vi "Edge Detection Comparizon.vi"() -> ()   [LabVIEW 2023]
doc: "This example shows the application of the wavelet transforms in detecting image edges.\n\nConventional edge detection methods process an image at a single resolution and return a binary edge map. The wavelet transform-based method processes an image at multiple levels of resolution and returns a series of grey-level edge maps at different resolutions. You can obtain the global profile of the image in a low-resolution edge map and the detailed texture of the image in a high-resolution edge map.\n\nThis example uses the WA Multiscale Edge Detection VI to detect the edges of an image.\n\n<b>Instructions:</b>\n1) Run this VI.\n2) Increase the value of <b>Level</b> to observe coarser edges.\n3) Increase the value of <b>Threshold Ratio</b> to skip the edges in darker areas."
uses:
  Images/_Images.ctl
  <vilib>/vision/NI_Vision_Development_Module.lvlib
panel:
  out "Edges 2":T1(plugin-control)
  in  "Threshold Value":sgl format="%.2f"
  in  "Method":T2(ring)
  out "error out":errorcluster
  in  "error in (no error)":errorcluster
  in  "Image":T3
  in  "wavelet":u16(ring)=20 items=["db02"=0, "db03"=1, "db04"=2, "db05"=3, "db06"=4, "db07"=5, "db08"=6, "db09"=7, "db10"=8, "db11"=9, "db12"=10, "db13"=11, "db14"=12, "Haar"=13, "bior1_3"=14, "bior1_5"=15, "bior2_2"=16, "bior2_4"=17, "bior2_6"=18, "bior2_8"=19, "bior3_1"=20, "bior3_3"=21, "bior3_5"=22, "bior3_7"=23, "bior3_9"=24, "bior4_4 (FBI)"=25, "bior5_5"=38, "bior6_8"=39, "coif1"=26, "coif2"=27, "coif3"=28, "coif4"=29, "coif5"=30, "sym2"=31, "sym3"=32, "sym4"=33, "sym5"=34, "sym6"=35, "sym7"=36, "sym8"=37]
  out "Edges":T1(plugin-control)
  out "Source Image":T1(plugin-control)
  in  "Level":i32=1 min=1 max=8
  in  "Threshold ratio":dbl=0.1 min=0.0001 max=1.0 step=0.1
  # "Edges detection using Wavelets"
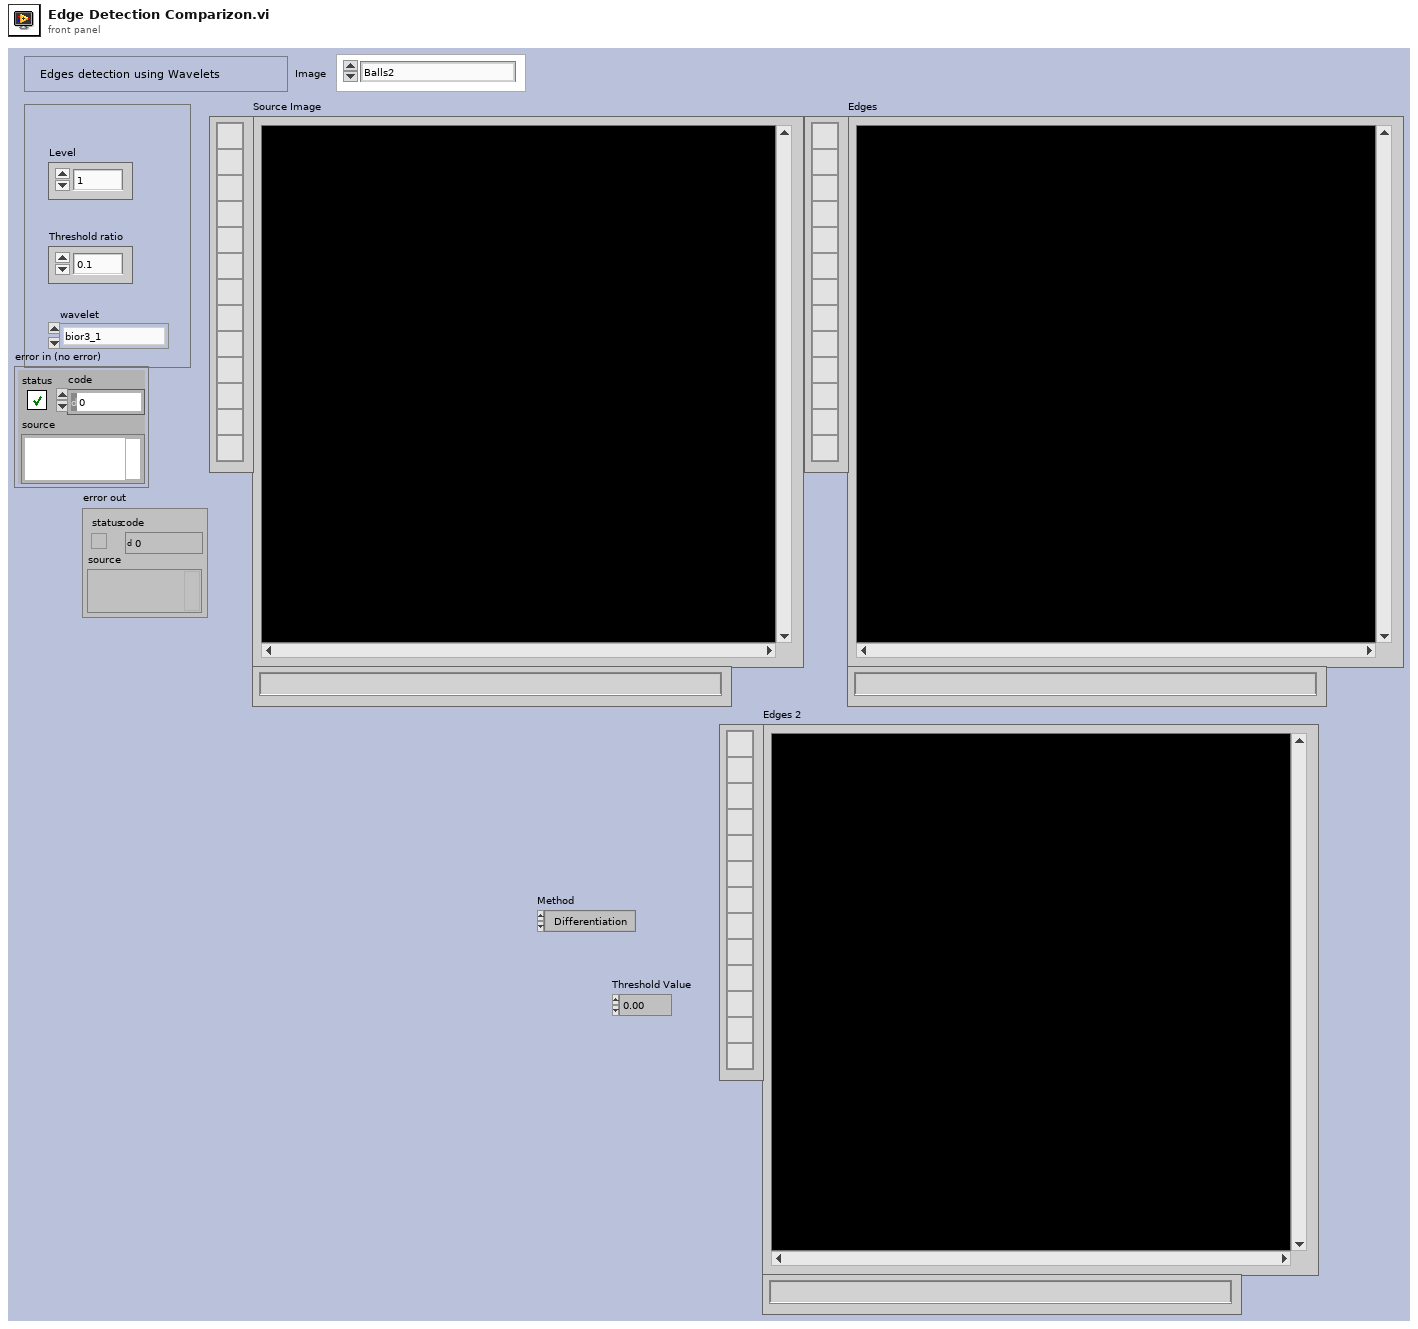
[diagram p1: front panel]
types:
  T1 = typedef "IMAQ Image.ctl" = refnum<image>
  T2 = enum32{"Differentiation", "Gradient", "Prewitt", "Roberts", "Sigma", "Sobel"}
  T3 = typedef "_Images.ctl" = enum16{"Balls2", "Battery1", "Battery2", "Connector1", "Subwoofer1", "Subwoofer2", "Subwoofer3", "Subwoofer4", "Hase1", "Lamp1", "Lamp2", "Mouse1", "PhotoLens1", "Po1", "PowerSupply1", "Router", "--- Step Wedges ---", "Stepwedge1", "Stepwedge2", "Stepwedge3", "--- Fusion ---", "Fusion160kV", "Fusion2-120kV", "Fusion2-320kV", "Fusion300kV", "FusionPart1-120kV", "FusionPart1-180kV", "--- PART 01 ---", "Part1", "Part2", "Part3", "Part4", "Part5", "Part6", "Part7", "Part8", "--- Different Integrations ---", "Step2737-02Int", "Step2737-04Int", "Step2737-08Int", "Step2737-16Int", "Step2737-32Int", "Step2737-64Int"}
  T4 = typedef "Image Type" = u32
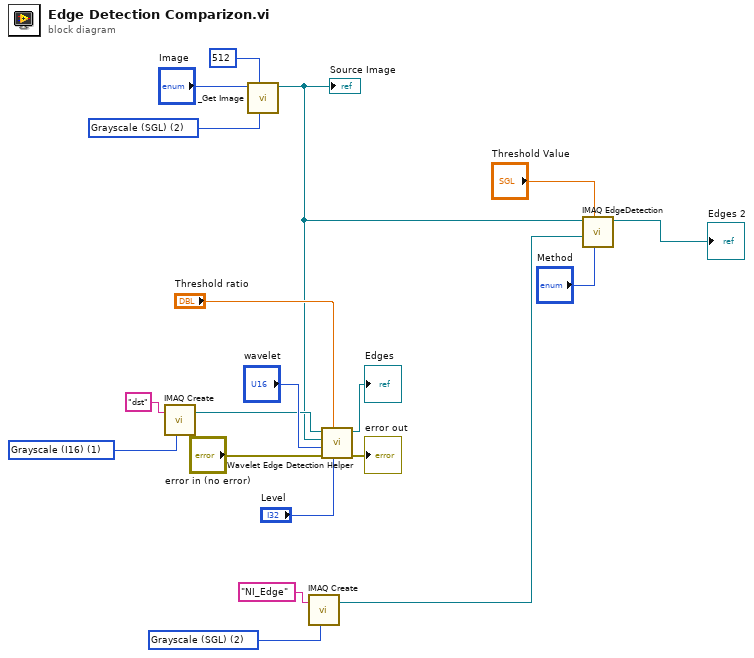
[diagram p0: block diagram]
diagram:
  w5 = T4 2 items=["Grayscale (U8)", "Grayscale (I16)", "Grayscale (SGL)", "Complex (CSG)", "RGB (U32)", "HSL (U32)", "RGB (U64)", "Grayscale (U16)"] ("Image Type")
  w14 = T4 1 items=["Grayscale (U8)", "Grayscale (I16)", "Grayscale (SGL)", "Complex (CSG)", "RGB (U32)", "HSL (U32)", "RGB (U64)", "Grayscale (U16)"] ("Image Type")
  w15 = T4 2 items=["Grayscale (U8)", "Grayscale (I16)", "Grayscale (SGL)", "Complex (CSG)", "RGB (U32)", "HSL (U32)", "RGB (U64)", "Grayscale (U16)"] ("Image Type (U16)")
  n1 = call "IMAQ Create"("Image Name"="dst", "Image Type"=w14) -> ("New Image"=w12:T1)  [unwired: 3 in, 1 out]
  n2 = call "_Get Image.vi"("Image Type (U16)"=w15, "XY Resolution"=512, "Image"="Image") -> ("Image Out"=w7:T1)  [unwired: 5 in, 3 out]
  "Source Image" <- w7
  n3 = call "IMAQ Create"("Image Name"="NI_Edge", "Image Type"=w5) -> ("New Image"=w1:T1)  [unwired: 3 in, 1 out]
  n4 = call "Wavelet Edge Detection Helper.vi"("Level"="Level", "Threshold ratio"="Threshold ratio", "error in (no error)"="error in (no error)", "wavelet"="wavelet", "Image In"=w7, "Refnum in"=w12) -> ("error out"=→"error out":errorcluster, "Refnum out"=→"Edges":T1)  [unwired: 3 in, 1 out]
  n5 = call "IMAQ EdgeDetection"("Method"="Method", "Threshold Value"="Threshold Value", "Image Dst"=w1, "Image Src"=w7) -> ("Image Dst Out"=→"Edges 2":T1)  [unwired: 6 in, 1 out]
